vi "imageSettings.vi"() -> ()   [LabVIEW 2016]
uses:
  <userlib>/atmcd64d.llb/HSSpeed_type typedef.ctl
panel:
  in  "realYDimension":dbl
  in  "stepLength":u32
  in  "realXDimension":dbl
  out "referenceExist":bool
  out "backgroundExist":bool
  out "hsArray":cluster{"String":string, "Value":u16}[](array[cluster])
  out "vsArray":cluster{"String":string, "Value":u16}[](array[cluster])
  in  "specArray":sgl[](array[numeric])
  in  "vss":i32
  in  "gainType":T1=enum."Conventional Amp"
  in  "hss":i32
  in  "Exposure Time (s)":sgl=0.01 step=0.001 format="%.4f"
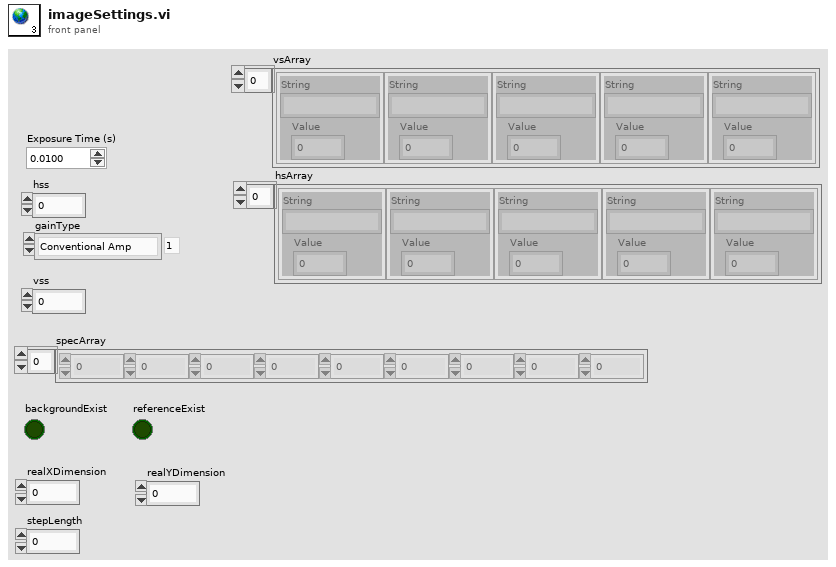
[diagram p1: front panel]
types:
  T1 = typedef "HSSpeed_type typedef.ctl" = enum16{"EM Amp", "Conventional Amp"}
diagram:
